vi "Abort Job.vi"(6 "timeout (500 ms)":i32=500, 8 "error in (no error)":errorcluster, 11 "Job in":refnum<class "Job.lvclass">) -> (0 "error out":errorcluster, 1 "Job Not running":bool, 2 "Job Aborted":bool, 3 "Job out":refnum<class "Job.lvclass">, 5 "exception":i32)   [LabVIEW 2013, in "openCronJob.lvlib" / "Job.lvclass"]
uses:
  Job.lvclass
  Job.lvclass/Job.ctl
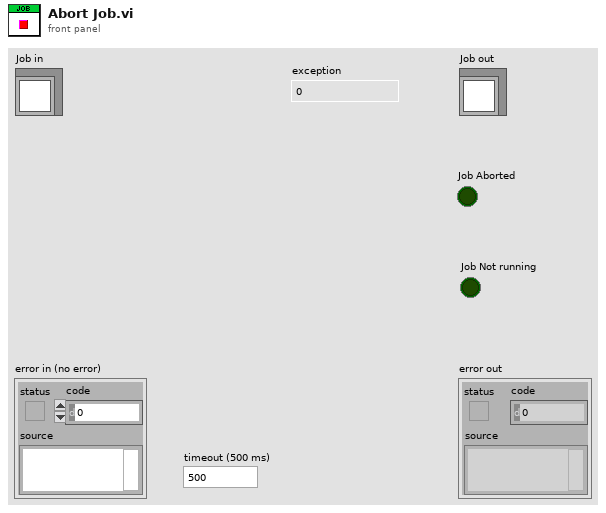
[diagram p1: front panel]
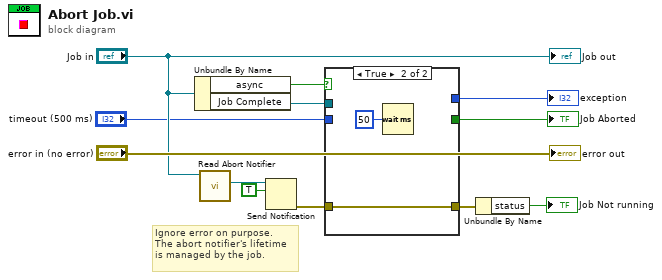
[diagram p0: block diagram]
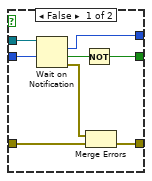
[diagram p2: hidden frame]
diagram:
  # "Ignore error on purpose.\nThe abort notifier's lifetime\nis managed by the job."
  n1 = Unbundle By Name("Job in") -> ("async"=w1:bool, "Job Complete"=w7:refnum<notifier>)
  n2 = call "Read Abort Notifier.vi"("Job in"="Job in") -> ("Abort"=w11:refnum<notifier>)  [unwired: 10 in]
  n3 = Send Notification(notification=TRUE, notifier=w11) -> (error out=w3:errorcluster)  [unwired: 1 in, 1 out]
  n4 = case shown="True" w1 {
    tunnel: w7 -> [w20 _]
    tunnel: "timeout (500 ms)" -> [w19 _]
    tunnel: [w17 _] -> w5
    tunnel: [w16 _] -> w4
    tunnel: w3 -> [w14 w22]
    tunnel: [w13 w22] -> w2
    frame False {
      n5 = Wait on Notification(notifier=w20, timeout in ms (-1)=w19) -> (notification=w16:i32, timed out?=w18:bool, error out=w15:errorcluster)  [unwired: 2 in, 1 out]
      n6 = Not(x=w18) -> (.not. x?=w17:bool)
      n7 = Merge Errors(w15, w14) -> (w13:errorcluster)
    }
    frame True {
      n8 = Wait (ms)(milliseconds to wait=u32 50) -> ()  [unwired: 1 out]
    }
  }
  "Job Aborted" <- w5
  "exception" <- w4
  n9 = Unbundle By Name(w2) -> ("status"=→"Job Not running":bool)
  "error out" <- "error in (no error)"
  "Job out" <- "Job in"
